vi "XIPIN_AXI_Central_Direct_Memory_Access_4_1.vi"   [LabVIEW 2017]
doc: "The AXI CDMA provides high-bandwidth direct memory access (DMA) between a memory mapped source address and a memory mapped destination address using the AXI4 protocol. An optional Scatter Gather (SG) feature can be used to offload control and sequencing tasks from the System CPU. Initialization, status, and control registers are accessed through an AXI4-Lite slave interface.\n------------------------------------\n<b>Need License</b> : No\n<b>Interface</b> : AXI4"
uses:
  <vilib>/rvi/XilinxIP/XIPIN_XNode/niFpgaXIPIN.xnode
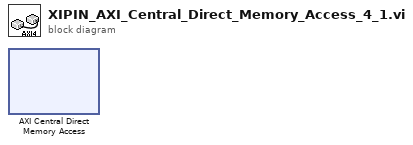
[diagram p0: block diagram]
diagram:
  n1 = xnode ("AXI Central Direct Memory Access")() -> ()
